vi "Read Connect Ref.vi"(8 "error in (no error)":errorcluster, 11 "ZanClass in":refnum<class "ZanClass.lvclass">) -> (0 "error out":errorcluster, 1 "Visa":string, 2 "CardHandle":i32, 3 "ZanClass out":refnum<class "ZanClass.lvclass">)   [LabVIEW 2019, in "ZanClass.lvclass"]
uses:
  ZanClass.lvclass
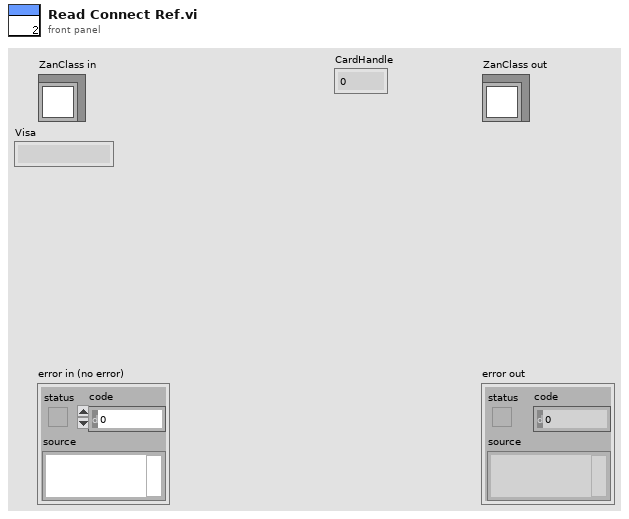
[diagram p1: front panel]
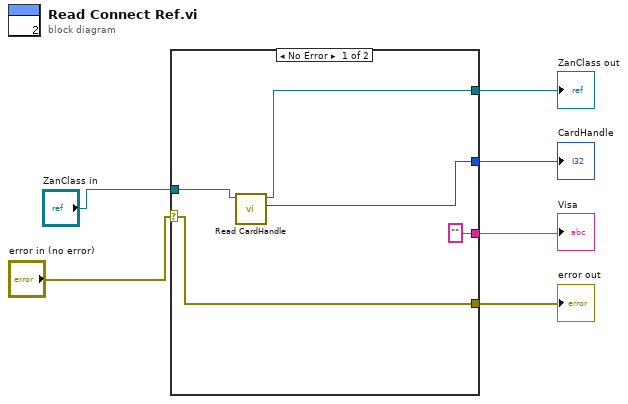
[diagram p0: block diagram]
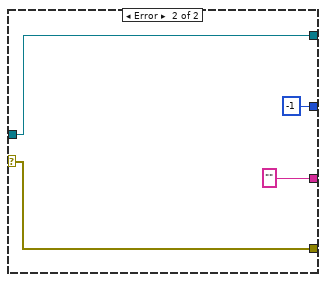
[diagram p2: hidden frame]
diagram:
  n1 = case shown="No Error" "error in (no error)" {
    selector: "error in (no error)" -> [w8 w12]
    tunnel: "ZanClass in" -> [w11 w15]
    tunnel: [w10 w15] -> w4
    tunnel: [w9 -1 ("CardHandle")] -> w3
    tunnel: ["" ""] -> w2
    tunnel: [w8 w12] -> w1
    frame No Error {
      n2 = call-dynamic "Read CardHandle.vi"("AxisCard in"=w11) -> ("CardHandle"=w9:i32, "AxisCard out"=w10:refnum<class "ZanClass.lvclass">)  [unwired: 8 in, 1 out]
    }
    frame Error {
    }
  }
  "error out" <- w1
  "ZanClass out" <- w4
  "Visa" <- w2
  "CardHandle" <- w3
